vi "twoAnalog_triggerAndStaircase_pyDLL_subVI.vi"(1 "zRage":dbl=5.0, 3 "Number of zPlanes":i32=15, 4 "Initial step {V}":dbl, 5 "delay [ms]":dbl, 6 "Max Voltage":dbl=5.0, 7 "triggerTiming [ms]":dbl=1.0, 10 "Min Voltage":dbl=-5.0, 11 "TTL uptime [%]":i32=50, 16 "Cluster":T1={"Physical Channel(s)"="Dev1/ao0:1", "Min Voltage"=-5.0, "Max Voltage"=5.0, "Sample Clock Source"="OnboardClock", "Number of zPlanes"=15, "zRage"=5.0, "Initial step {V}"=0.0, "amplitude TTL [V]"=5.0, "triggerTiming [ms]"=1.0, "Number of Points per step (must be even)"=1000, "TTL uptime [%]"=25, "delay [ms]"=0.0}) -> (13 "message":string="No Error", 14 "sawArray":dbl[](array[numeric]), 15 "trigArray":dbl[](array[numeric]), 17 "Array":cluster{dbl[], "initialized array":dbl[]}[](array[cluster]), 18 "number of samples written per channel":u32=15000, 19 "code out":i32)   [LabVIEW 2020]
uses:
  <vilib>/Utility/error.llb/DialogType.ctl
  <vilib>/DAQmx/write.llb/DAQmx Write (Analog 2D DBL NChan NSamp).vi
  <vilib>/DAQmx/create/channels.llb/DAQmx Create Channel (AO-Voltage-Basic).vi
  <vilib>/DAQmx/configure/timing.llb/DAQmx Timing (Sample Clock).vi
  <vilib>/DAQmx/miscellaneous.llb/DAQmx Fill In Error Info.vi
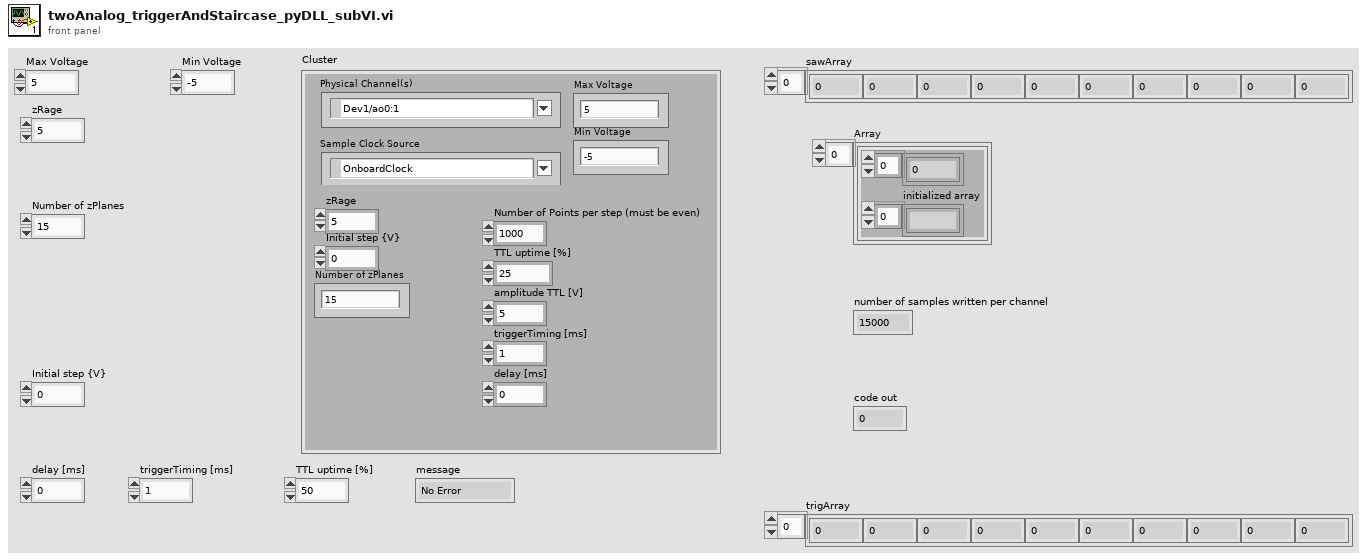
[diagram p1: front panel]
types:
  T1 = cluster{"Physical Channel(s)":tag, "Min Voltage":dbl, "Max Voltage":dbl, "Sample Clock Source":tag, "Number of zPlanes":i32, "zRage":dbl, "Initial step {V}":dbl, "amplitude TTL [V]":dbl, "triggerTiming [ms]":dbl, "Number of Points per step (must be even)":i32, "TTL uptime [%]":i32, "delay [ms]":dbl}
  T2 = typedef "DialogType.ctl" = u16
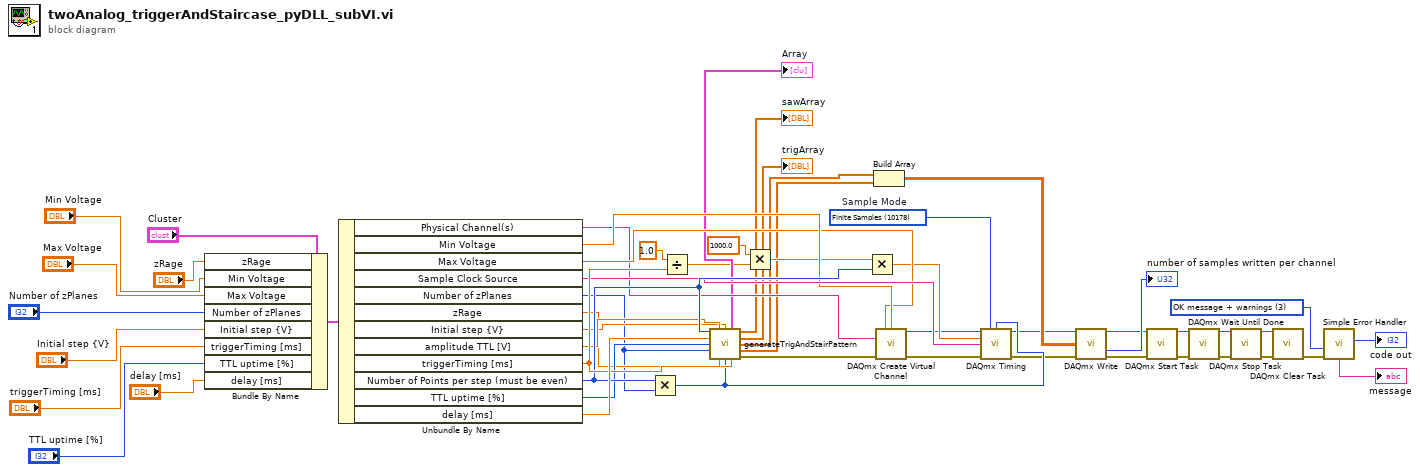
[diagram p0: block diagram]
diagram:
  w12 = T2 3 items=["no dialog", "OK message", "continue or stop message", "OK message + warnings", "continue/stop + warnings"] ("type of dialog (OK msg:1)")
  w13 = 10178 items=["Finite Samples"=10178, "Continuous Samples"=10123, "Hardware Timed Single Point"=12522]  # Sample Mode
  n1 = Bundle By Name(cluster="Cluster", "zRage"="zRage", "Min Voltage"="Min Voltage", "Max Voltage"="Max Voltage", "Number of zPlanes"="Number of zPlanes", "Initial step {V}"="Initial step {V}", "triggerTiming [ms]"="triggerTiming [ms]", "TTL uptime [%]"="TTL uptime [%]", "delay [ms]"="delay [ms]") -> (w42:T1)
  n2 = Unbundle By Name(w42) -> ("Physical Channel(s)"=w29:tag, "Min Voltage"=w31:dbl, "Max Voltage"=w30:dbl, "Sample Clock Source"=w32:tag, "Number of zPlanes"=w33:i32, "zRage"=w34:dbl, "Initial step {V}"=w35:dbl, "amplitude TTL [V]"=w36:dbl, "triggerTiming [ms]"=w39:dbl, "Number of Points per step (must be even)"=w38:i32, "TTL uptime [%]"=w37:i32, "delay [ms]"=w40:dbl)
  n3 = Multiply(x=w38, y=w33) -> (x*y=w22:i32)
  n4 = Divide(x=1.0, y=w39) -> (x/y=w17:dbl)
  n5 = call "generateTrigAndStairPattern.vi"("Number of Points per step (must be even)"=w38, "amplitude TTL [V]"=w36, "Initial step {V}"=w35, "delay [ms]"=w40, "TTL uptime [%]"=w37, "Number of zPlanes"=w33, "triggerTiming [ms]"=w39, "Numeric"=w22, "zRage"=w34) -> ("Array"=→"Array":cluster{dbl[], "initialized array":dbl[]}[], "sawArray"=→"sawArray":dbl[], "trigArray"=→"trigArray":dbl[], "initialized array 2"=w20:dbl[], "initialized array"=w23:dbl[], "error out"=w41:errorcluster)  [unwired: 1 in]
  n6 = Multiply(x=1000.0, y=w17) -> (x*y=w25:dbl)
  n7 = Multiply(x=w25, y=w38) -> (x*y=w26:dbl)
  n8 = Build Array(w20, w23) -> (w19:dbl[][])
  n9 = call-poly <vilib>:"DAQmx Create Virtual Channel.vi"("maximum value"=w30, "minimum value"=w31, "physical channels"=w29, "error in"=w41) -> ("task out"=w2:refnum<k21>, "error out"=w1:errorcluster)  [unwired: 10 in]
  n10 = call-poly <vilib>:"DAQmx Timing.vi"("task/channels in"=w2, "sample mode"=w13, "samples per channel"=w22, "rate"=w26, "source"=w32, "error in"=w1) -> ("task out"=w14:refnum<k21>, "error out"=w15:errorcluster)  [unwired: 8 in]
  n11 = call-poly <vilib>:"DAQmx Write.vi"("task/channels in"=w14, "data"=w19, "error in"=w15) -> ("task out"=w4:refnum<k21>, "number of samples written per channel"=→"number of samples written per channel":u32, "error out"=w5:errorcluster)  [unwired: 10 in]
  n12 = call <vilib>:"DAQmx Start Task.vi"("task/channels in"=w4, "error in"=w5) -> ("task out"=w6:refnum<k21>, "error out"=w7:errorcluster)  [unwired: 12 in]
  n13 = call <vilib>:"DAQmx Wait Until Done.vi"("task/channels in"=w6, "error in"=w7) -> ("task out"=w10:refnum<k21>, "error out"=w11:errorcluster)  [unwired: 12 in]
  n14 = call <vilib>:"DAQmx Stop Task.vi"("task/channels in"=w10, "error in"=w11) -> ("task out"=w8:refnum<k21>, "error out"=w9:errorcluster)  [unwired: 12 in]
  n15 = call <vilib>:"DAQmx Clear Task.vi"("task in"=w8, "error in"=w9) -> ("error out"=w3:errorcluster)  [unwired: 13 in]
  n16 = call <vilib>:"Simple Error Handler.vi"("type of dialog (OK msg:1)"=w12, "error in (no error)"=w3) -> ("code out"=→"code out":i32, "message"=→"message":string)  [unwired: 3 in, 3 out]
